vi "Car Position.vi"(10 "Position Needed":T1(ring), 11 "Car Position Slider":u8(slide) max=3 scale=0.0..4.0) -> (3 "In Position":bool)   [LabVIEW 2018]
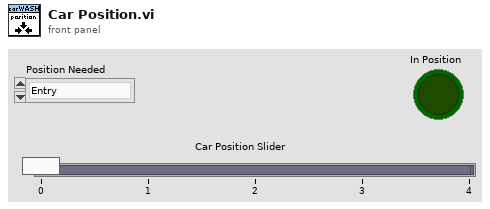
[diagram p1: front panel]
types:
  T1 = enum16{"Entry", "Station 1", "Station 2", "Station 3", "Exit"}
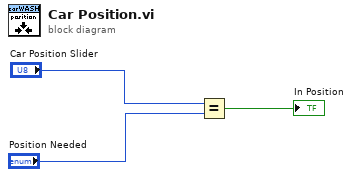
[diagram p0: block diagram]
diagram:
  n1 = Equal?(x="Car Position Slider", y="Position Needed") -> (x = y?=→"In Position":bool)
